vi "Verzoegerung PC.vi"(7 "Abfallverzögerung?":bool, 8 "ms":u16, 9 "sec":u16, 10 "min":u16, 11 "Startsignal":bool) -> (0 "Aktuelle Zeit [sec]":sgl, 3 "Zeit abgelaufen?":bool)   [LabVIEW 2020, in "allgemeine Sub-VIs.lvlib"]
uses:
  allgemeine Sub-VIs.lvlib
panel:
  # "VI Einstellung:\nAblaufinvarinate Ausführung\nKopie für jede Instanz vorbelegen\n(behält Zustand für jede Instanz bei)"
  # "PC"
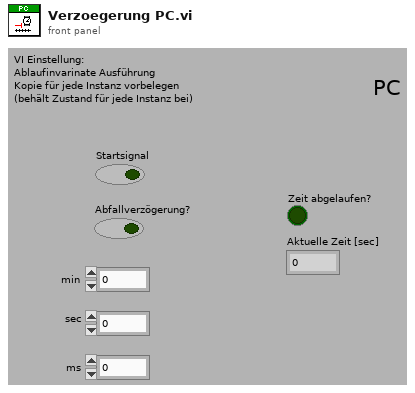
[diagram p1: front panel]
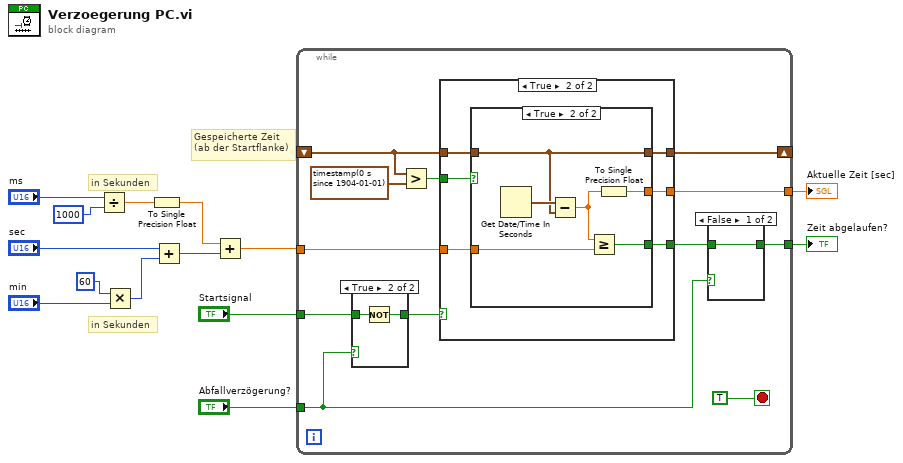
[diagram p0: block diagram]
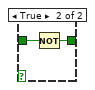
[diagram p2: hidden frame]
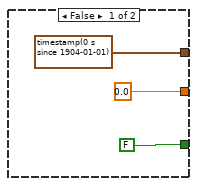
[diagram p4: hidden frame]
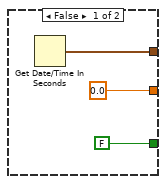
[diagram p5: hidden frame]
diagram:
  # "in Sekunden"
  # "in Sekunden"
  # "Gespeicherte Zeit\n(ab der Startflanke)"
  n1 = Divide(x="ms", y=u16 1000) -> (x/y=w3:dbl)
  n2 = Multiply(x=u16 60 ("y"), y="min") -> (x*y=w10:u16)
  n3 = To Single Precision Float(number=w3) -> (single precision float=w2:sgl)
  n4 = Add(x="sec", y=w10) -> (x+y=w6:u16)
  n5 = Add(x=w2, y=w6) -> (x+y=w5:sgl)
  n6 = while {
    shift-right: [w25] -> _
    shift-left: _ -> [w24]
    tunnel: w5 -> [w22]
    tunnel: "Startsignal" -> [w17]
    tunnel: [w21] -> w13
    tunnel: "Abfallverzögerung?" -> [w18]
    tunnel: [w15] -> w1
    stop <- TRUE stop-if-true
    n7 = case shown="True" w18 {
      tunnel: w17 -> [w30 w32]
      tunnel: [w30 w31] -> w16
      frame False {
      }
      frame True {
        n8 = Not(x=w32) -> (.not. x?=w31:bool)
      }
    }
    n9 = Greater?(x=w24, y=timestamp(0 s since 1904-01-01) ("Aktuelle Zeit")) -> (0:w23:bool)
    n10 = case shown="True" w16 {
      tunnel: [timestamp(0 s since 1904-01-01) ("Aktuelle Zeit") w41] -> w25
      tunnel: w24 -> [_ w39]
      tunnel: w23 -> [_ w40]
      tunnel: w22 -> [_ w38]
      tunnel: [FALSE w37] -> w19
      tunnel: [sgl 0.0 w36] -> w21
      frame False {
      }
      frame True {
        n11 = case shown="True" w40 {
          tunnel: [w44 w48] -> w41
          tunnel: w39 -> [_ w48]
          tunnel: w38 -> [_ w49]
          tunnel: [FALSE w47] -> w37
          tunnel: [sgl 0.0 w46] -> w36
          frame False {
            n12 = Get Date/Time In Seconds() -> (seconds since 1Jan1904=w44:timestamp)
          }
          frame True {
            n13 = Get Date/Time In Seconds() -> (seconds since 1Jan1904=w50:timestamp)
            n14 = Subtract(x=w50, y=w48) -> (x-y=w45:dbl)
            n15 = Greater Or Equal?(x=w45, y=w49) -> (x >= y?=w47:bool)
            n16 = To Single Precision Float(number=w45) -> (single precision float=w46:sgl)
          }
        }
      }
    }
    n17 = case shown="False" w18 {
      tunnel: w19 -> [w27 w29]
      tunnel: [w27 w28] -> w15
      frame False {
      }
      frame True {
        n18 = Not(x=w29) -> (.not. x?=w28:bool)
      }
    }
  }
  "Zeit abgelaufen?" <- w1
  "Aktuelle Zeit [sec]" <- w13
